vi "Measurement UI.vi"() -> ()   [LabVIEW 2021, in "Single Tone No Gen_Class D Amplifier_UI.lvlib"]
uses:
  Single Tone No Gen_Class D Amplifier_UI.lvlib
  shared/controls/units - snr.ctl
  shared/controls/units - ratio.ctl
  shared/ui/controls/view.ctl
  UI State.ctl
  <vilib>/Utility/miscctls.llb/LVBoundsTypeDef.ctl
  <vilib>/Utility/miscctls.llb/LVPoint32TypeDef.ctl
  <vilib>/Utility/miscctls.llb/LVPointTypeDef.ctl
  shared/ui/UI Helpers.lvlib
  shared/controls/audio controls.lvlib
panel:
  in  "view legend":T1
  out "time domain":waveform(dbl)[](graph)
  out "frequency domain":cluster{"x0":dbl, "dx":dbl, "magnitude":dbl[]}[](graph)
  out "meas table":string[][](table)
  out "output power (W)":dbl[](array[numeric])
  out "SFDR (dBc)":dbl[](array[numeric])
  out "gain":dbl[](array[numeric])
  out "dynamic range (dB)":dbl[](array[numeric])
  out "THD":dbl[](array[numeric])
  out "THD+N":dbl[](array[numeric])
  out "SNR":dbl[](array[numeric])
  out "phase (deg)":dbl[](array[numeric])
  out "amplitude (dBFS)":dbl[](array[numeric])
  out "amplitude (Vrms)":dbl[](array[numeric])
  out "frequency (Hz)":dbl[](array[numeric])
  out "channel names":string[](array[string])
  in  "Configuration tab":enum32{"Measurement", "Units"}(tab)
  in  "expected amplitude (Vpk)":dbl=1000.0 caption="Expected amplitude" format="%#_6f Vpk"
  in  "min settling cycles":u32 caption="Minimum settling cycles"
  in  "min settling time (s)":dbl=0.1 caption="Minimum settling time" format="%#_6ps"
  in  "min measurement cycles":u32 caption="Minimum measurement cycles"
  in  "min measurement time (s)":dbl=0.1 caption="Minimum measurement time" format="%#_6ps"
  in  "Acquisition channel":tag
  in  "acq sampling rate":dbl=51200.0 caption="Sample rate" format="%#.6pHz"
  in  "lowpass filter":T2(ring) caption="Lowpass filter"
  in  "highpass filter":enum32{"DC", "AC"}(ring) caption="Highpass filter"
  in  "band start":dbl=20.0 caption="Band start" format="%#_6pHz"
  in  "band stop":dbl=20000.0 caption="Band stop" format="%#_6pHz"
  in  "weighting filter":T3(ring)=enum."A-weighting" caption="Weighting filter"
  in  "load impedance":dbl=4.0 caption="Load impedance" format="%#_6p Ohms"
  in  "amplitude reference (Vpk-pk)":dbl=15.0 caption="Amplitude reference" format="%.3p Vpk-pk"
  in  "signal frequency":dbl=1000.0 caption="Estimated frequency" format="%#_6pHz"
  in  "gain units":T4 caption="Gain"
  in  "THD units":T4 caption="THD"
  in  "THD+N units":T4 caption="THD+N"
  in  "SNR units":T5 caption="SNR"
  in  "channel 0 offset":u32=1
  out "fft - data":dbl[](array[numeric])
  out "fft - df":dbl
  out "fft - f0":dbl
  out "wfm - data":dbl[](array[numeric])
  out "wfm - dt":dbl
  out "wfm - t0":dbl
  in  "acq channel":string="PXI1Slot4/ai0"
  in  "signal phase":dbl caption="phase"
  # "hidden controls - used to sync with MeasLink"
  # "hidden indicators"
  # "Filters"
  # "Acquisition"
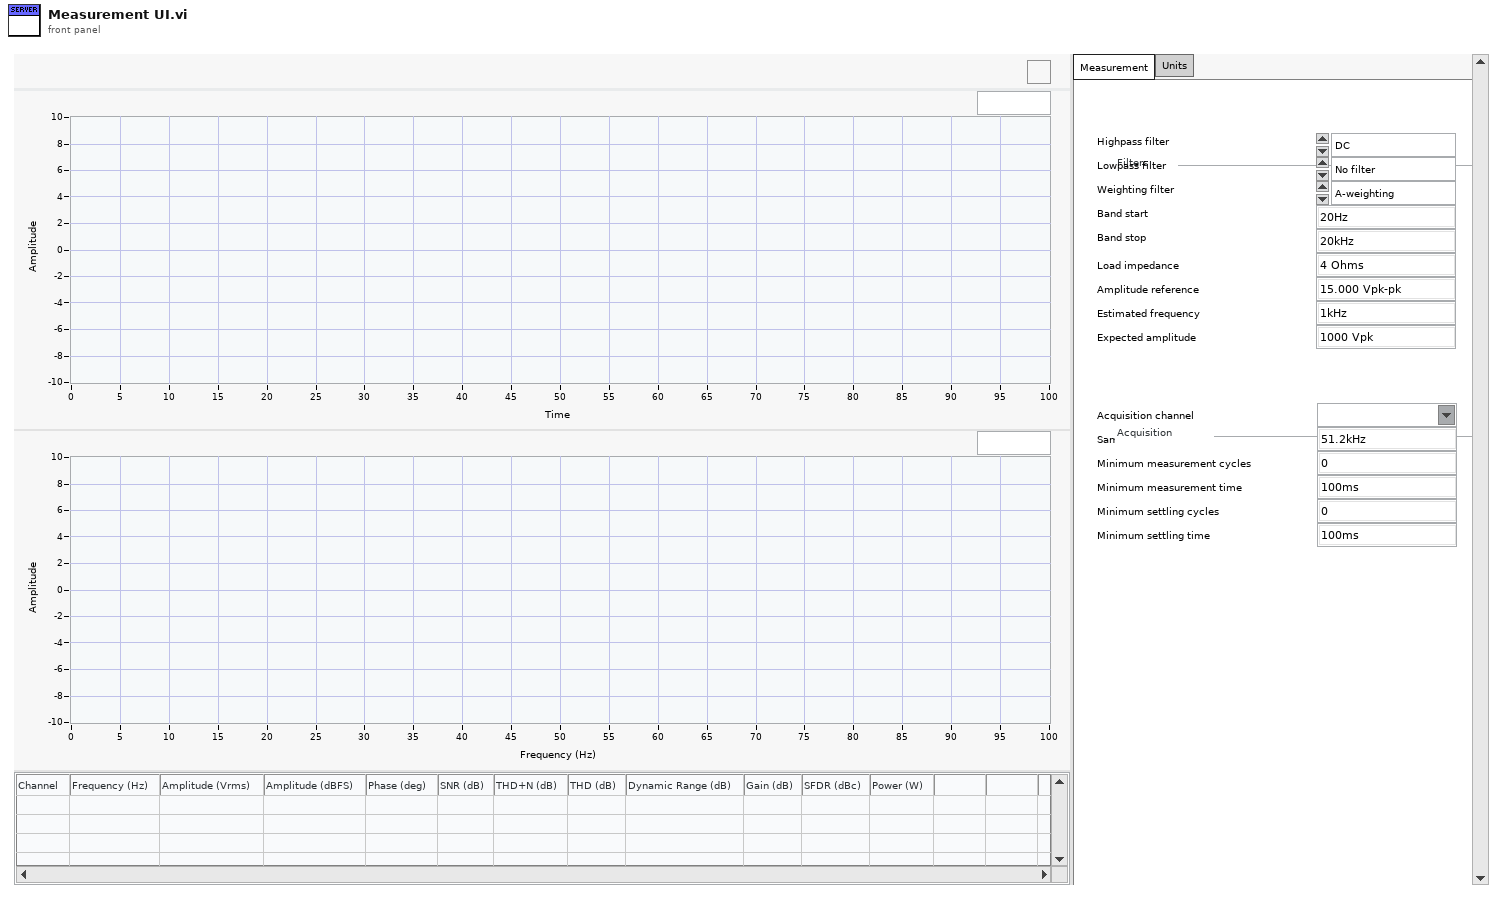
[diagram p1: front panel]
types:
  T1 = typedef "UI Helpers.lvlib/view.ctl" = bool
  T2 = enum32{"No filter", "AES17 20kHz", "AES17 40kHz"}
  T3 = enum32{"Linear", "A-weighting", "B-weighting", "C-weighting"}
  T4 = typedef "audio controls.lvlib/units - ratio.ctl" = enum32{"dB", "%", "x/y"}
  T5 = typedef "audio controls.lvlib/units - snr.ctl" = enum32{"dB", "x/y"}
  T6 = typedef "LVPointTypeDef.ctl" = cluster{"Horizontal":i16, "Vertical":i16}
  T7 = typedef "Single Tone No Gen_Class D Amplifier_UI.lvlib/UI State.ctl" = cluster{"Graph Size":T8, "Legend Visible":bool, "Mouse Coords":T9, "Show All Plots":bool}
  T8 = typedef "LVBoundsTypeDef.ctl" = cluster{"Width":u32, "Height":u32}
  T9 = typedef "LVPoint32TypeDef.ctl" = cluster{"Horizontal":i32, "Vertical":i32}
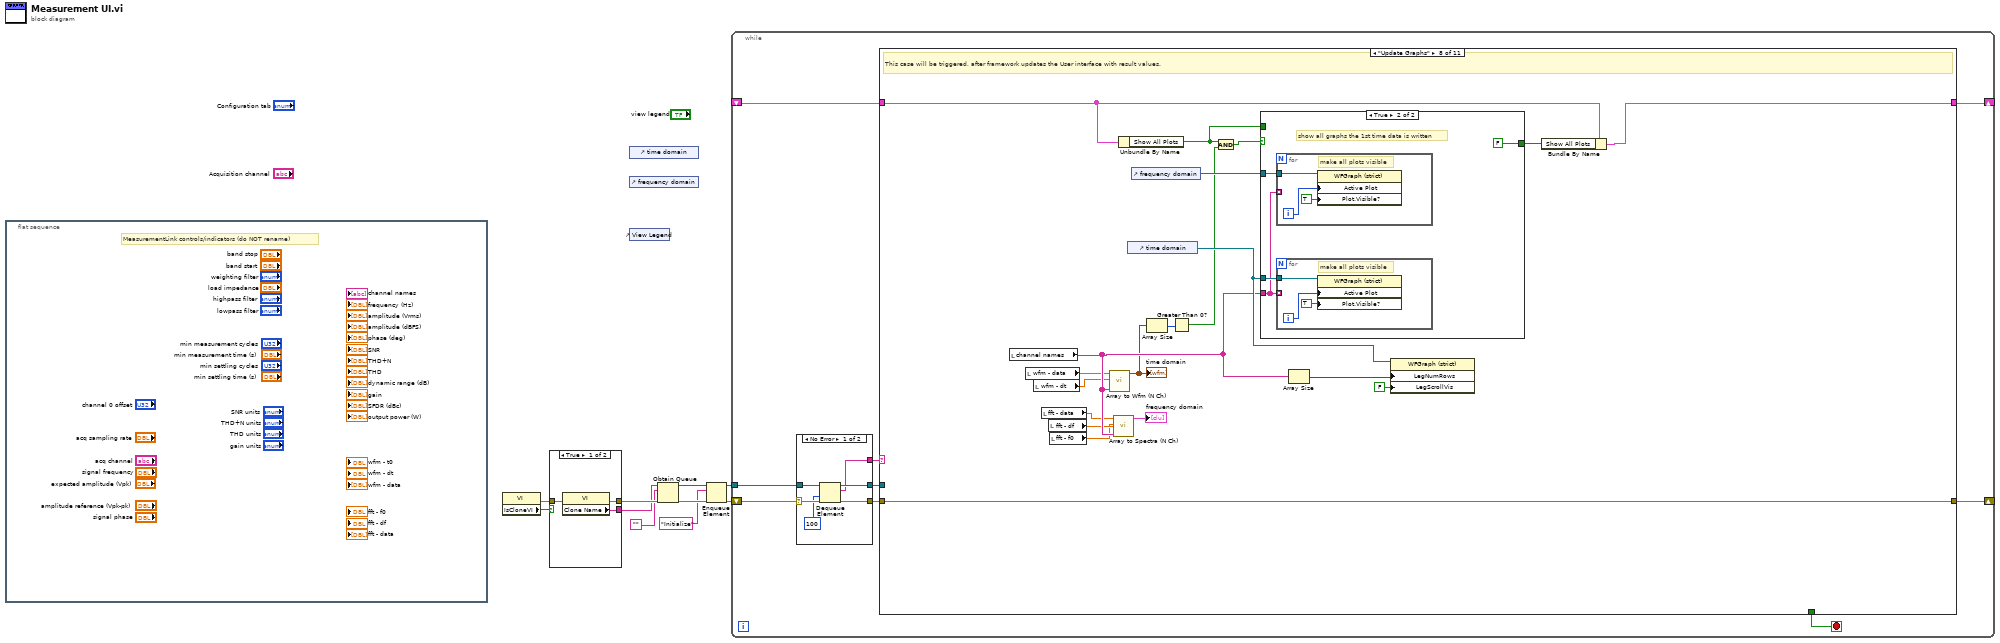
[diagram p0: block diagram]
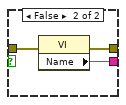
[diagram p2: hidden frame]
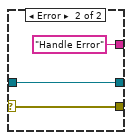
[diagram p3: hidden frame]
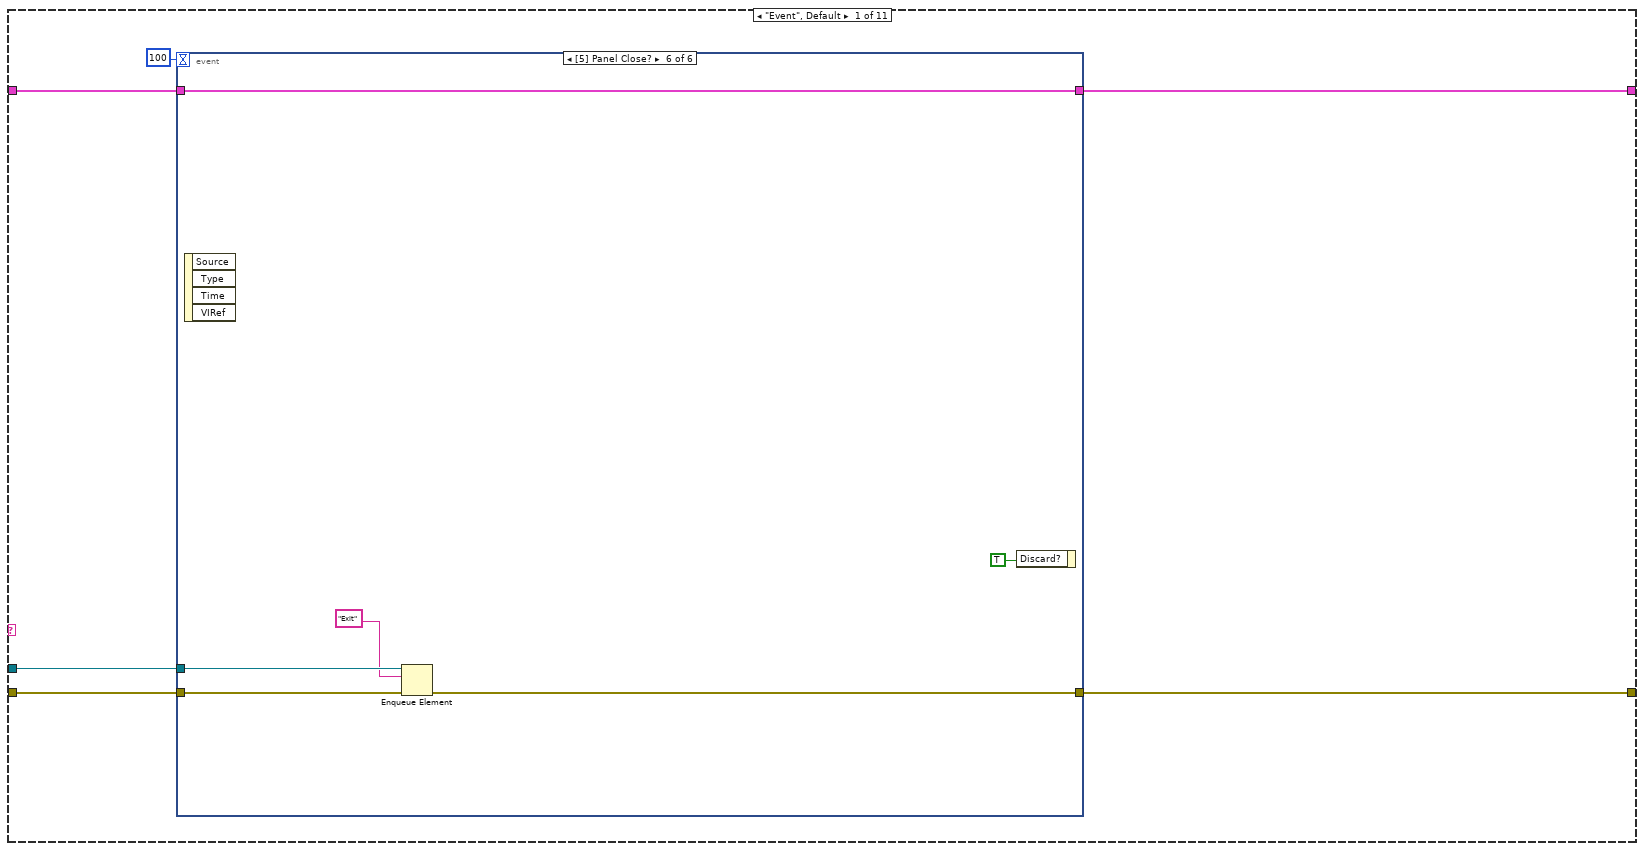
[diagram p4: hidden frame]
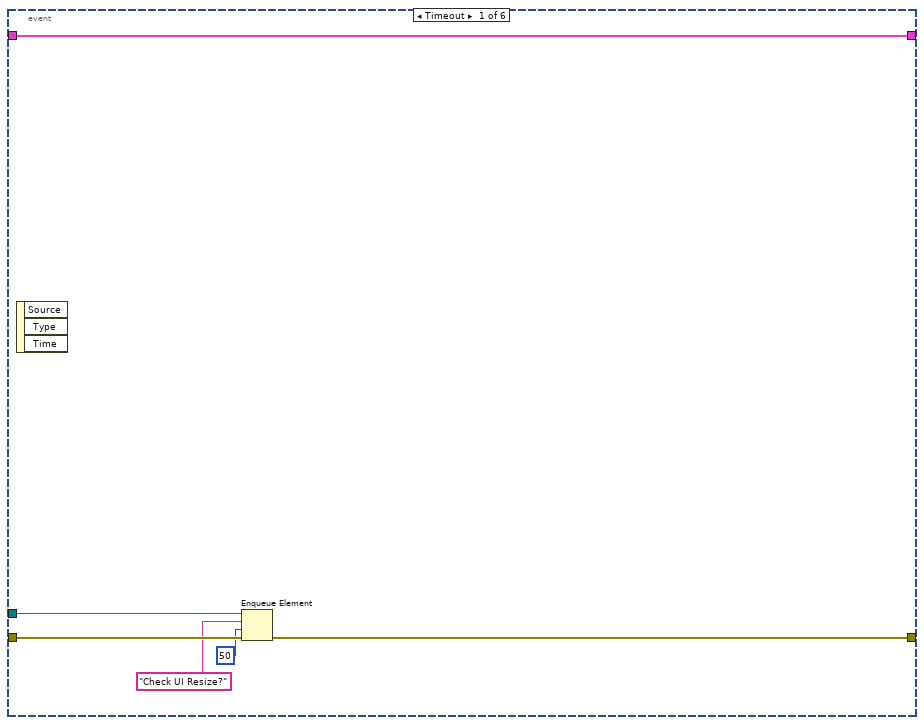
[diagram p5: hidden frame]
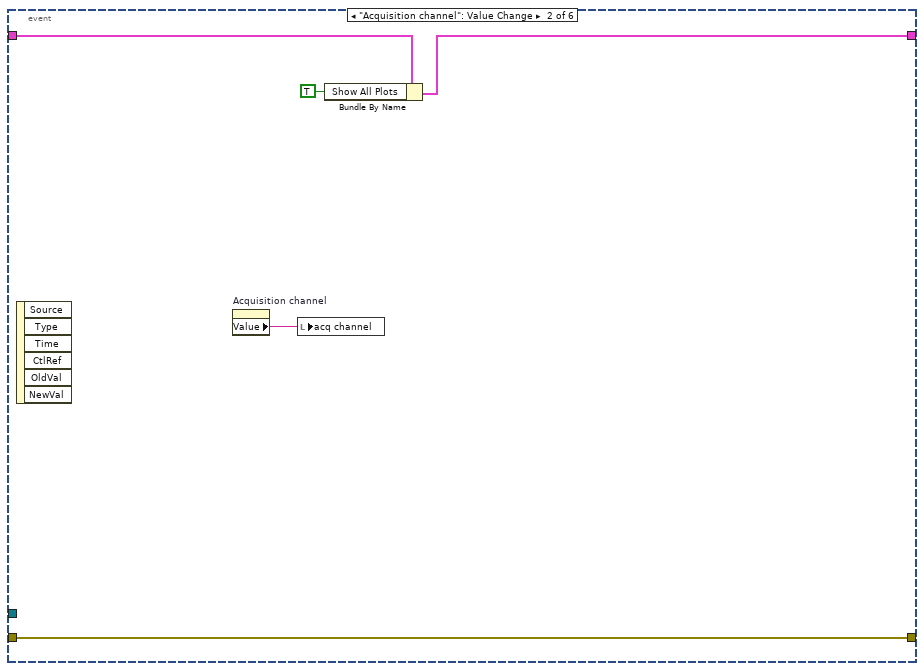
[diagram p6: hidden frame]
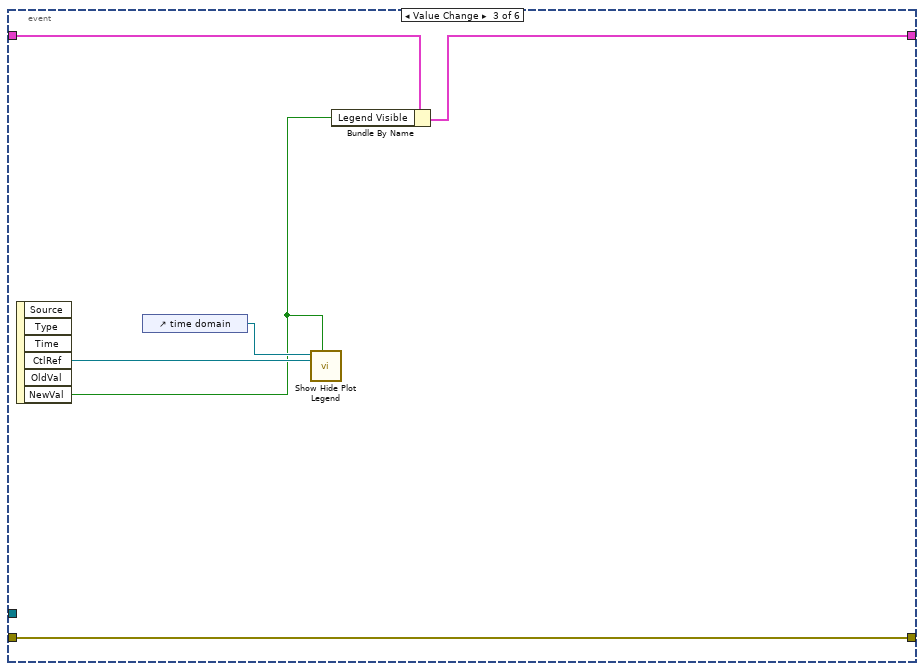
[diagram p7: hidden frame]
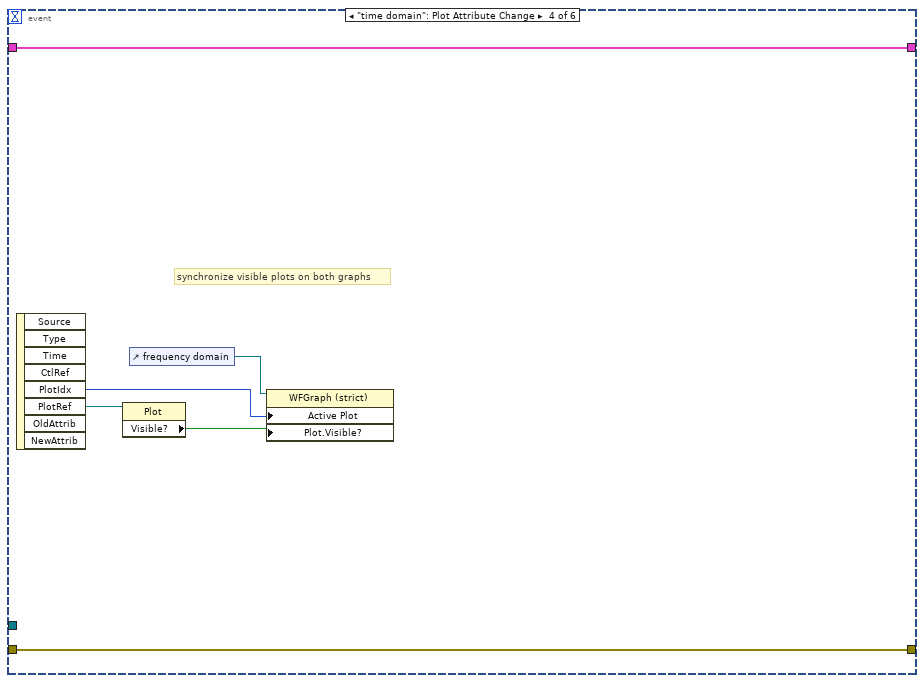
[diagram p8: hidden frame]
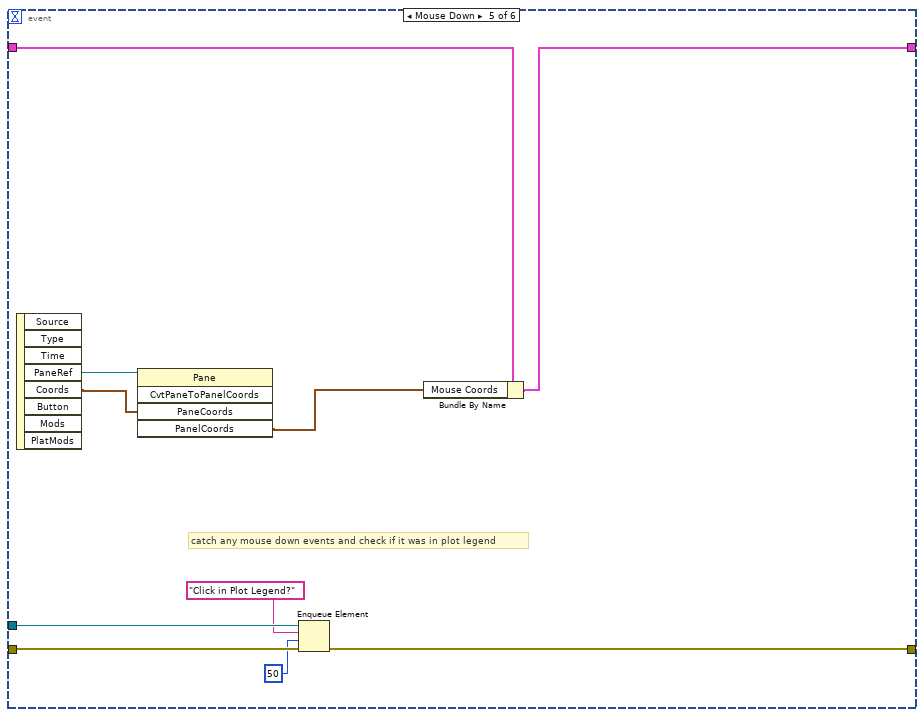
[diagram p9: hidden frame]
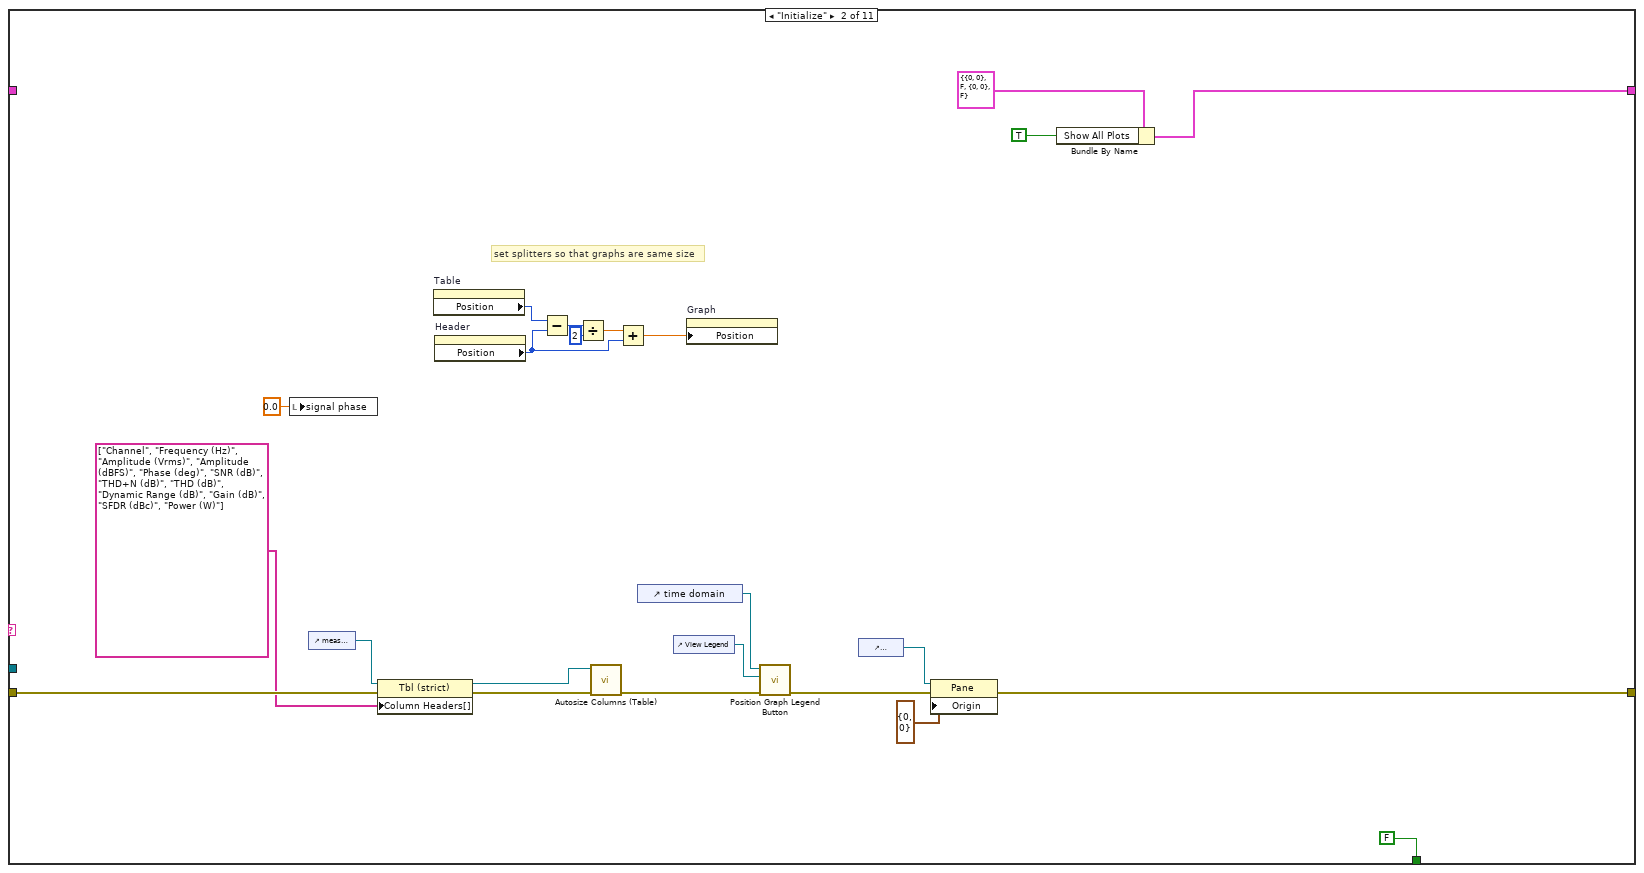
[diagram p10: hidden frame]
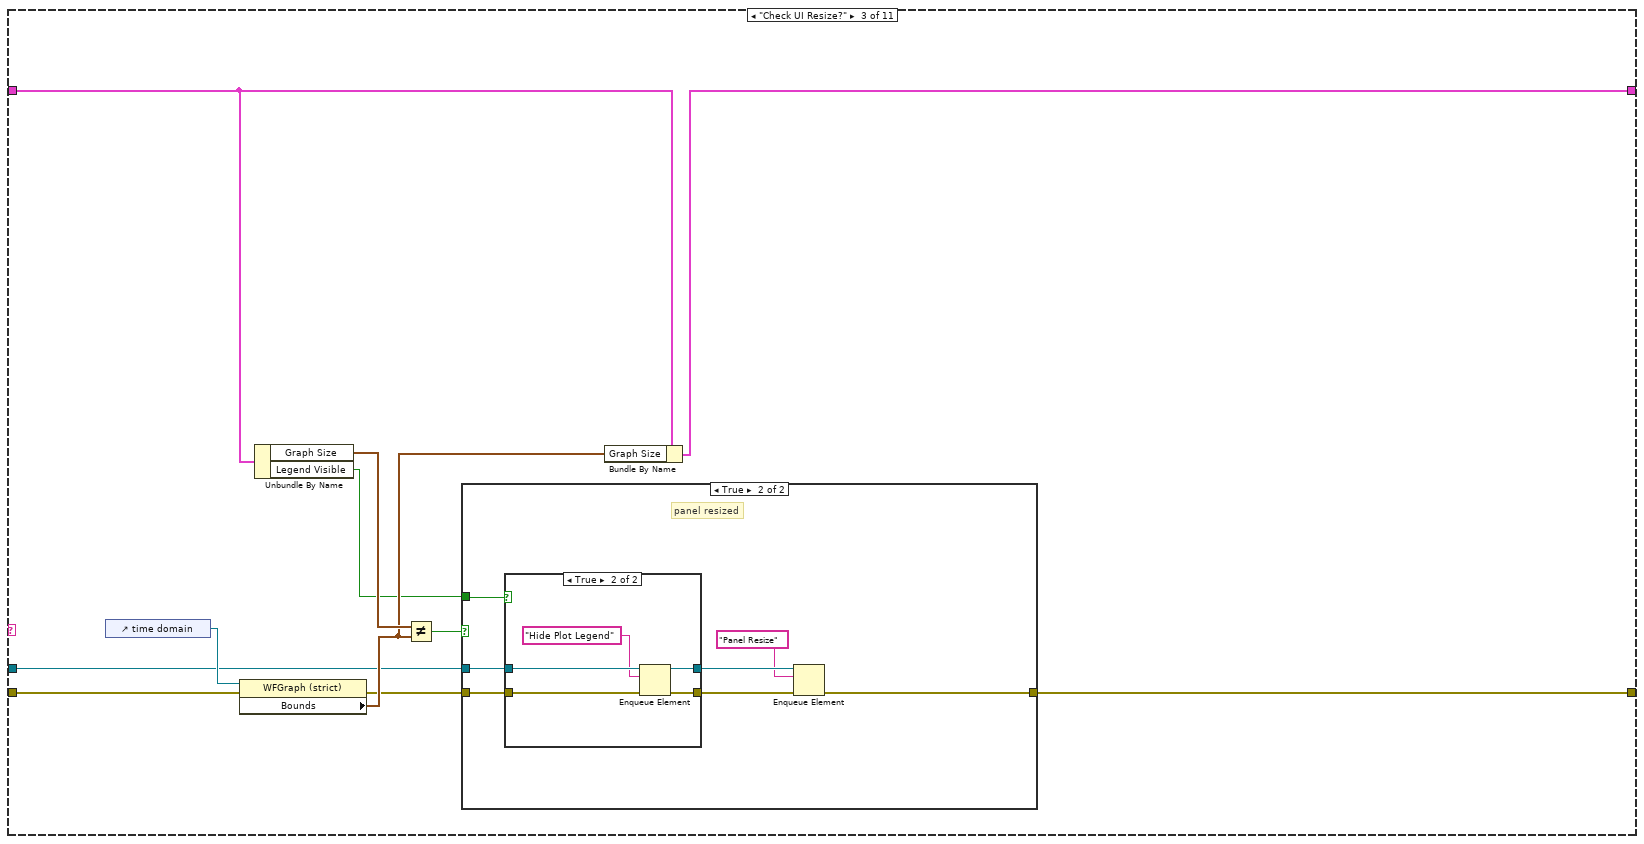
[diagram p11: hidden frame]
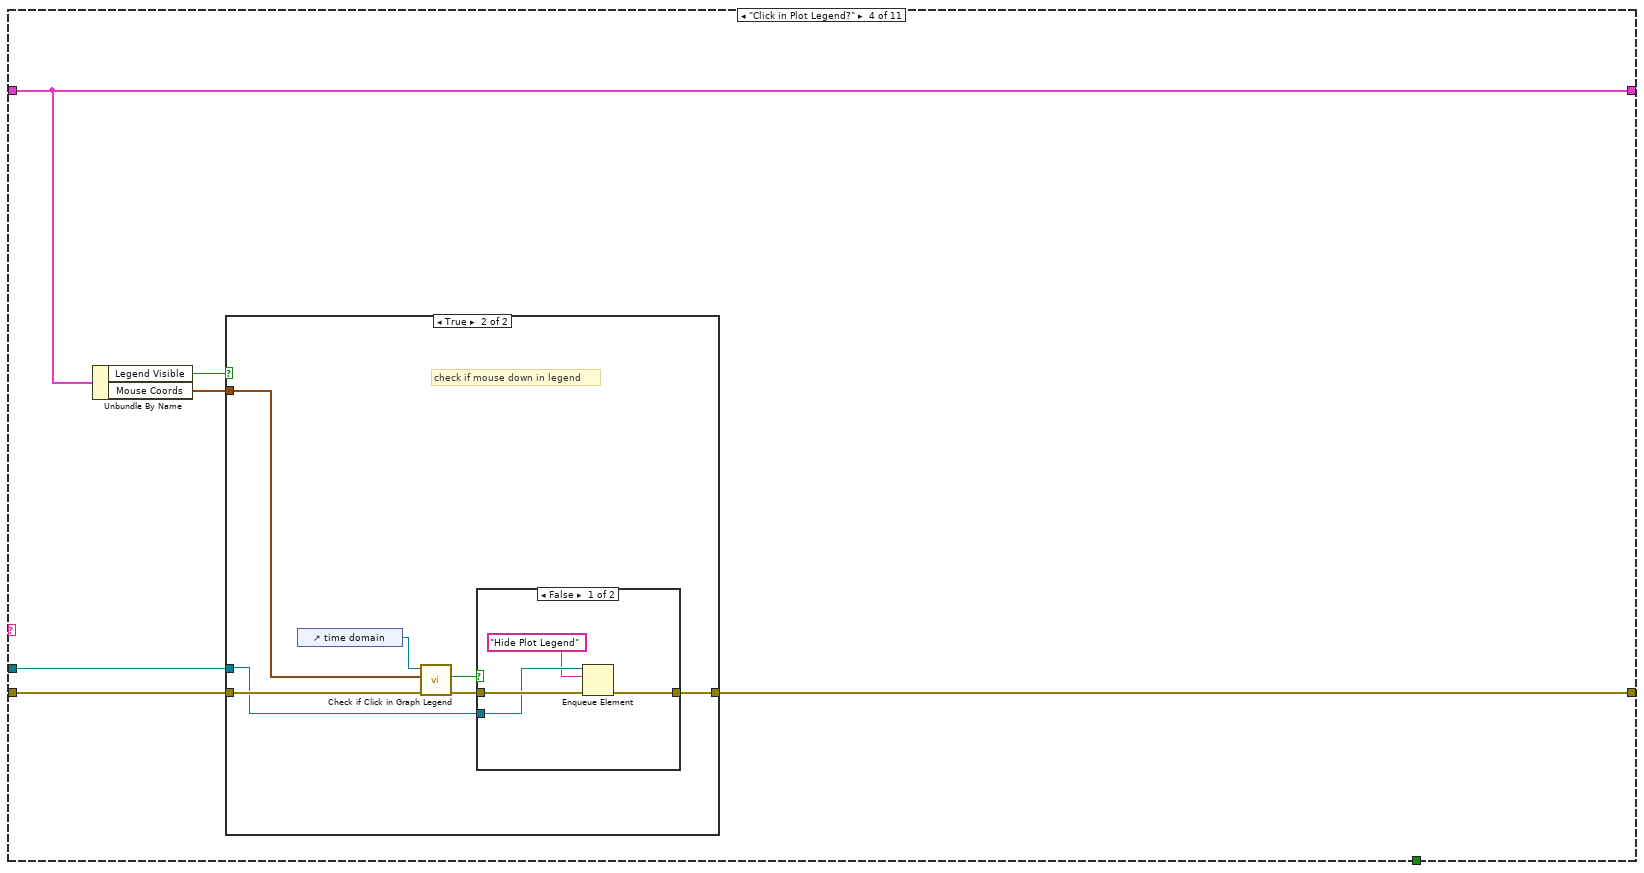
[diagram p14: hidden frame]
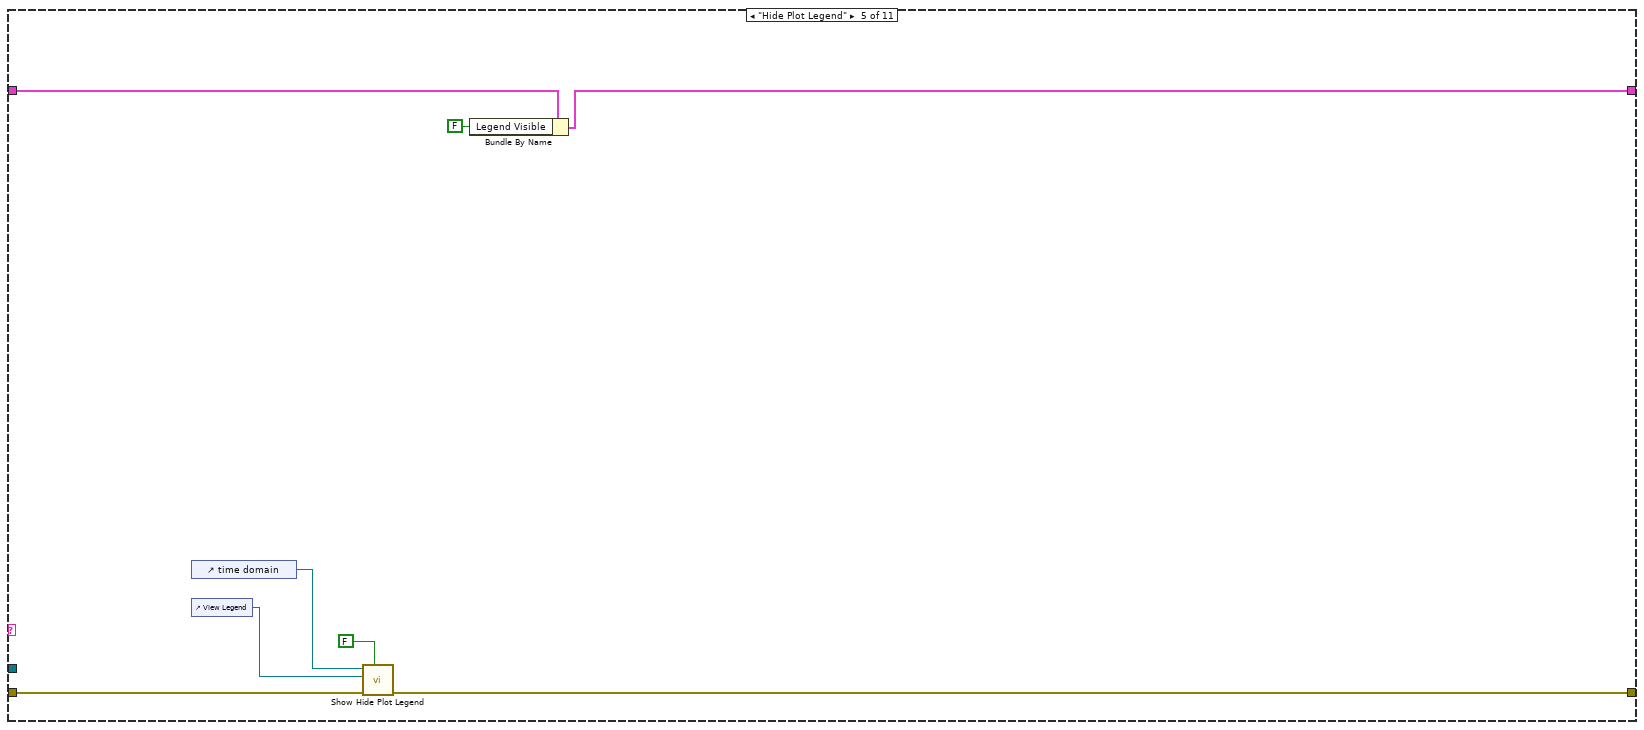
[diagram p17: hidden frame]
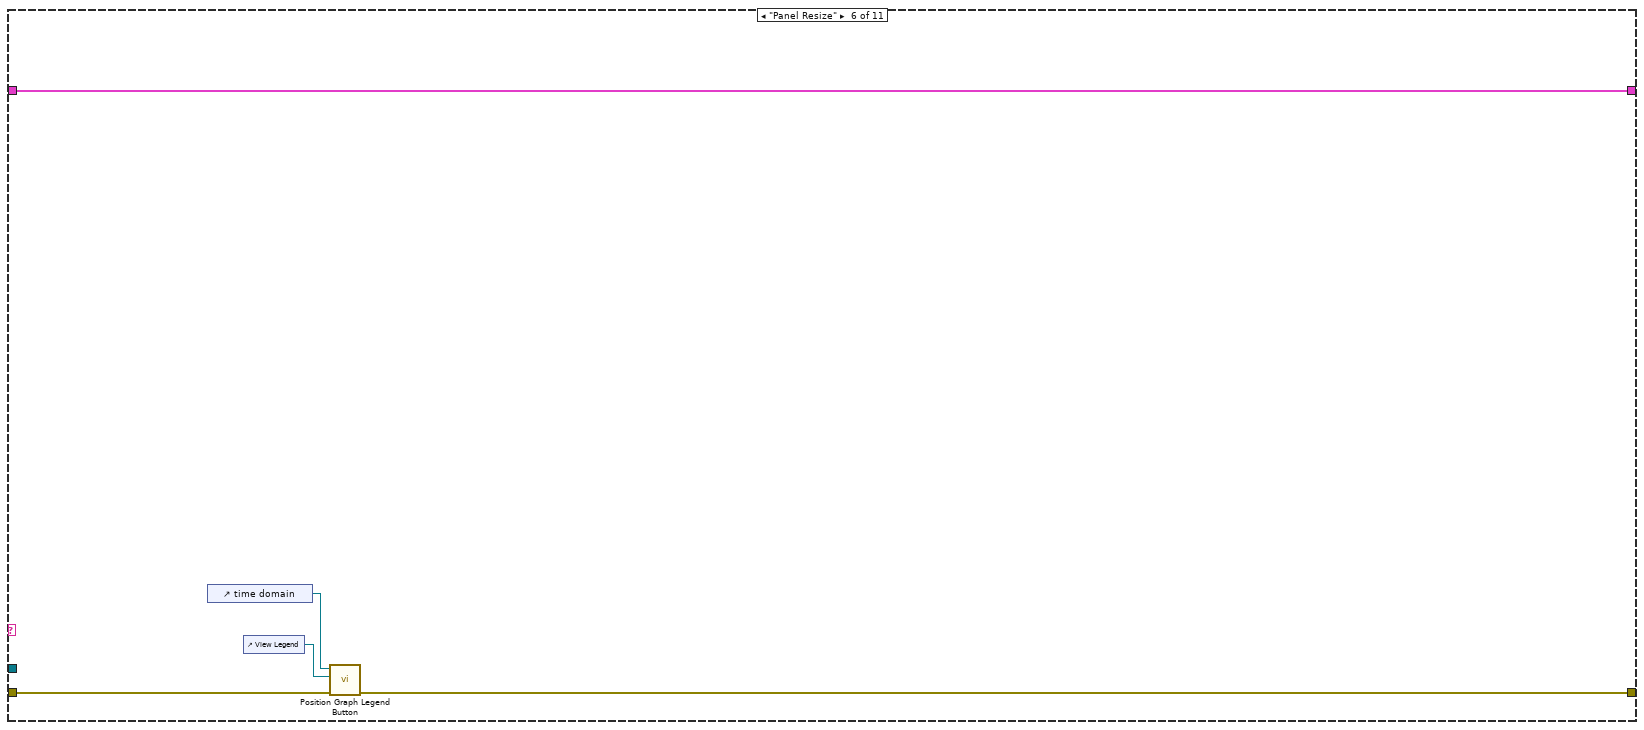
[diagram p18: hidden frame]
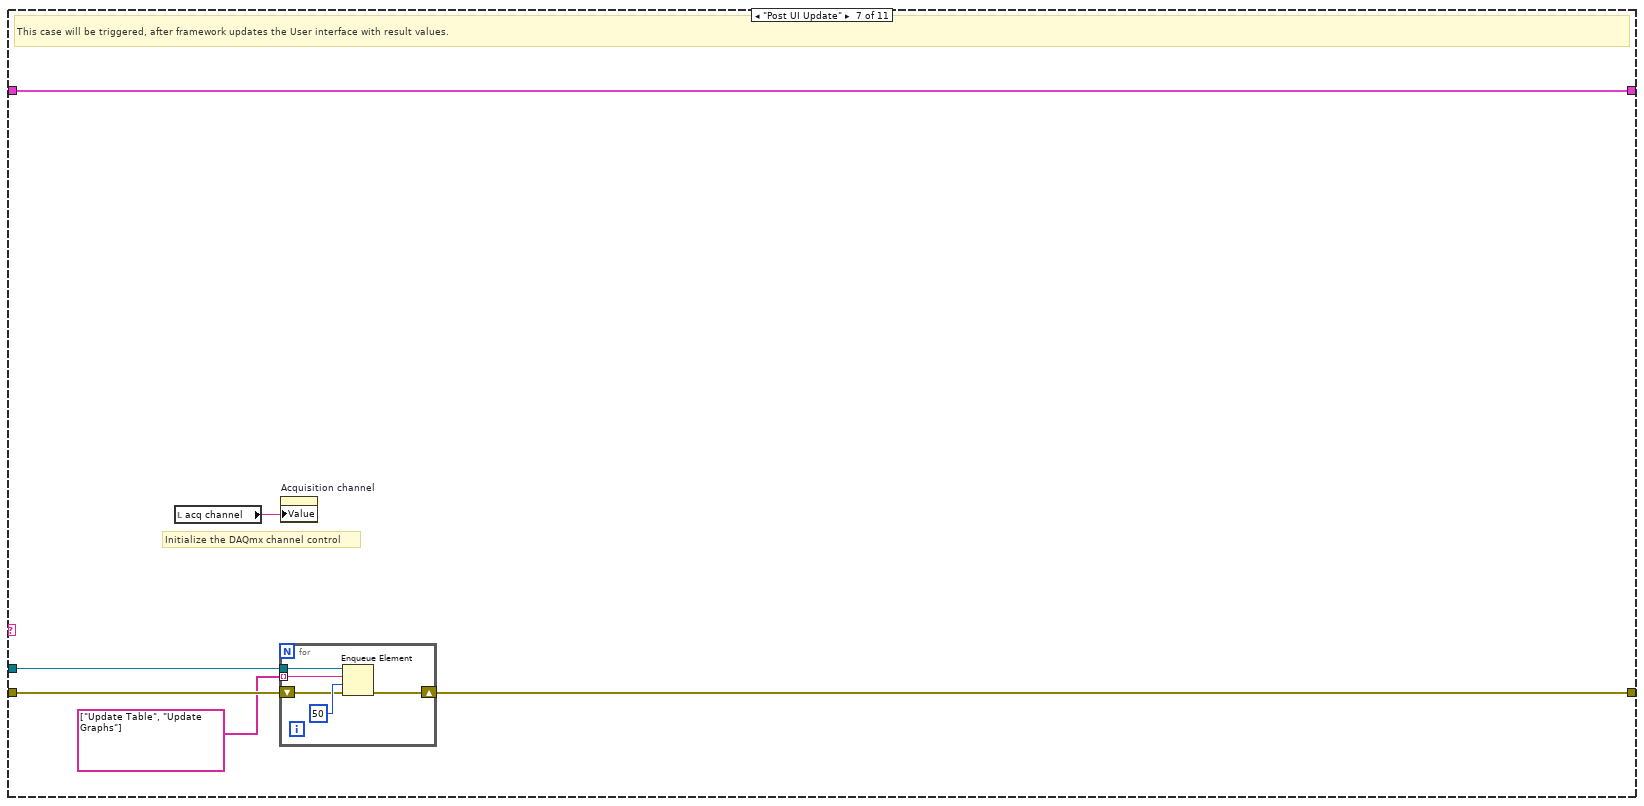
[diagram p19: hidden frame]
diagram:
  n1 = flat-sequence {
    frame #0 {
      # "MeasurementLink controls/indicators (do NOT rename)"
    }
  }
  n2 = property class="VI"() -> (error out=w1:errorcluster, "IsCloneVI"=w2:bool)  [unwired: 2 in, 1 out]
  n3 = case shown="True" w2 {
    tunnel: [w13 w16] -> w10
    tunnel: [w12 w15] -> w9
    tunnel: w1 -> [w11 w14]
    frame True {
      n4 = property class="VI"(error in=w11) -> (error out=w13:errorcluster, "Clone Name"=w12:string)  [unwired: 1 in, 1 out]
    }
    frame False {
      n5 = property class="VI"(error in=w14) -> (error out=w16:errorcluster, "Name"=w15:string)  [unwired: 1 in, 1 out]
    }
  }
  n6 = control-ref of="time domain"() -> ()  [unwired: 1 out]
  n7 = control-ref of="frequency domain"() -> ()  [unwired: 1 out]
  n8 = control-ref of="View Legend"() -> ()  [unwired: 1 out]
  n9 = Obtain Queue(name (unnamed)=w9, element data type="", error in (no error)=w10) -> (queue out=w6:refnum<queue>, error out=w8:errorcluster)  [unwired: 2 in, 1 out]
  n10 = Enqueue Element(queue=w6, element="Initialize", error in (no error)=w8) -> (queue out=w5:refnum<queue>, error out=w7:errorcluster)  [unwired: 1 in, 1 out]
  n11 = while {
    shift-right: [w20] -> _
    shift-left: w7 -> [w25]
    tunnel: w5 -> [w23]
    shift-right: [w18] -> _
    shift-left: _ -> [w17]
    stop <- w19 stop-if-true
    n12 = case shown="No Error" w25 {
      selector: w25 -> [w31 w34]
      tunnel: [w30 w34] -> w24
      tunnel: w23 -> [w29 w33]
      tunnel: [w28 w33] -> w22
      tunnel: [w27 "Handle Error"] -> w21
      frame No Error {
        n13 = Dequeue Element(queue=w29, timeout in ms (-1)=100, error in (no error)=w31) -> (queue out=w28:refnum<queue>, element=w27:string, error out=w30:errorcluster)  [unwired: 1 out]
      }
      frame Error {
      }
    }
    n14 = case shown="\"Update Graphs\"" w21 {
      tunnel: w24 -> [w39 w97 w112 w130 w152 w157 w164 w191 w203 w329 w331]
      tunnel: w22 -> [w37 _ w103 w131 _ _ w163 _ _ w327 _]
      tunnel: [w40 w80 w105 w129 w151 w156 w161 w191 w207 w324 w331] -> w20
      tunnel: [_ FALSE _ _ _ _ _ _ _ TRUE _] -> w19
      tunnel: [w35 w85 w108 w134 w153 w160 w165 w183 w204 w322 w330] -> w18
      tunnel: w17 -> [w36 _ w109 w134 w154 w160 w165 w184 w204 w322 w330]
      frame "Event", Default {
        n15 = event shown="[5] Panel Close?" {
          selector: _ -> [_ _ _ _ _ _]
          dyn-events: _ -> [_ _ _ _ _ _]
          timeout: 100 -> [_ _ _ _ _ _]
          tunnel: [w43 w50 w54 w58 w71 w77] -> w40
          tunnel: w39 -> [w46 w50 w54 w58 w72 w78]
          tunnel: w37 -> [w45 _ _ _ w73 w76]
          tunnel: w36 -> [w42 w49 w56 w59 w68 w74]
          tunnel: [w42 w48 w55 w59 w67 w74] -> w35
          event Timeout {
            n16 = event-data() -> ()  [unwired: 1 in, 3 out]
            n17 = Enqueue Element(queue=w45, element="Check UI Resize?", timeout in ms (-1)=50, error in (no error)=w46) -> (error out=w43:errorcluster)  [unwired: 2 out]
          }
          event "Acquisition channel": Value Change {
            n18 = event-data() -> ()  [unwired: 1 in, 6 out]
            n19 = property on="Acquisition channel" class="DAQmxName"() -> ("Value"=w51:string)  [unwired: 2 in, 2 out]
            n20 = local write "acq channel"(w51) -> ()
            n21 = Bundle By Name(cluster=w49, "Show All Plots"=TRUE) -> (w48:T7)
          }
          event Value Change {
            n22 = event-data() -> ("CtlRef"=w53:refnum<vi>, "NewVal"=w52:T1)  [unwired: 1 in, 4 out]
            n23 = control-ref of="time domain"() -> (w57:refnum<vi>)
            n24 = call "Show Hide Plot Legend.vi"("show"=w52, "view reference"=w53, "graph reference"=w57) -> ()  [unwired: 8 in, 1 out]
            n25 = Bundle By Name(cluster=w56, "Legend Visible"=w52) -> (w55:T7)
          }
          event "time domain": Plot Attribute Change {
            # "synchronize visible plots on both graphs"
            n26 = event-data() -> ("PlotIdx"=w61:i32, "PlotRef"=w62:refnum<vi>)  [unwired: 1 in, 6 out]
            n27 = property class="Plot"(reference=w62) -> ("Visible?"=w63:bool)  [unwired: 1 in, 2 out]
            n28 = control-ref of="frequency domain"() -> (w60:refnum<vi>)
            n29 = property on="Property Node" class="WFGraph (strict)"(reference=w60, "Active Plot"=w61, "Plot.Visible?"=w63) -> ()  [unwired: 1 in, 2 out]
          }
          event Mouse Down {
            # "catch any mouse down events and check if it was in plot legend"
            n30 = event-data() -> ("PaneRef"=w66:refnum<vi>, "Coords"=w65:T9)  [unwired: 1 in, 6 out]
            n31 = invoke class="Pane" method="CvtPaneToPanelCoords"(reference=w66, "PaneCoords"=w65) -> ("PanelCoords"=w64:T6)  [unwired: 3 in, 4 out]
            n32 = Enqueue Element(queue=w73, element="Click in Plot Legend?", timeout in ms (-1)=50, error in (no error)=w72) -> (error out=w71:errorcluster)  [unwired: 2 out]
            n33 = Bundle By Name(cluster=w68, "Mouse Coords"=w64) -> (w67:T7)
          }
          event Panel Close? {
            n34 = event-data() -> ()  [unwired: 1 in, 4 out]
            n35 = Enqueue Element(queue=w76, element="Exit", error in (no error)=w78) -> (error out=w77:errorcluster)  [unwired: 1 in, 2 out]
            n36 = event-data("Discard?"=TRUE) -> ()  [unwired: 1 in, 1 out]
          }
        }
      }
      frame "Initialize" {
        # "set splitters so that graphs are same size"
        n37 = local write "signal phase"(0.0 ("signal phase")) -> ()
        n38 = control-ref of="meas table"() -> (w95:refnum<vi>)
        n39 = property class="Tbl (strict)"(reference=w95, error in=w97, "Column Headers[]"=string[] ["Channel", "Frequency (Hz)", "Amplitude (Vrms)", "Amplitude (dBFS)", "Phase (deg)", "SNR (dB)", "THD+N (dB)", "THD (dB)", "Dynamic Range (dB)", "Gain (dB)", "SFDR (dBc)", "Power (W)"] ("Column Header Strings[]")) -> (reference out=w94:refnum<vi>, error out=w96:errorcluster)
        n40 = property on="Table" class="Splitter"() -> ("Position"=w92:i32)  [unwired: 2 in, 2 out]
        n41 = property on="Header" class="Splitter"() -> ("Position"=w88:i32)  [unwired: 2 in, 2 out]
        n42 = Subtract(x=w92, y=w88) -> (x-y=w91:i32)
        n43 = Divide(x=w91, y=2) -> (x/y=w89:dbl)
        n44 = call "Autosize Columns (Table).vi"("error in (no error)"=w96, "table"=w94) -> ("error out"=w98:errorcluster)  [unwired: 9 in]
        n45 = Add(x=w89, y=w88) -> (x+y=w87:dbl)
        n46 = control-ref of="time domain"() -> (w100:refnum<vi>)
        n47 = control-ref of="View Legend"() -> (w99:refnum<vi>)
        n48 = property on="Graph" class="Splitter"("Position"=w87) -> ()  [unwired: 2 in, 2 out]
        n49 = call "Position Graph Legend Button.vi"("error in (no error)"=w98, "view legend"=w99, "graph"=w100) -> ("error out"=w83:errorcluster)  [unwired: 8 in]
        n50 = control-ref of="Configuration"() -> (w82:refnum<vi>)
        n51 = property class="Pane"(reference=w82, error in=w83, "Origin"=T6 {"Horizontal"=0, "Vertical"=0}) -> (error out=w80:errorcluster)  [unwired: 1 out]
        n52 = Bundle By Name(cluster=T7 {"Graph Size"={"Width"=0, "Height"=0}, "Legend Visible"=FALSE, "Mouse Coords"={"Horizontal"=0, "Vertical"=0}, "Show All Plots"=FALSE} ("ui state"), "Show All Plots"=TRUE ("Init Graph Plot Legend")) -> (w85:T7)
      }
      frame "Check UI Resize?" {
        n53 = control-ref of="time domain"() -> (w113:refnum<vi>)
        n54 = property on="Property Node" class="WFGraph (strict)"(reference=w113, error in=w112) -> (error out=w106:errorcluster, "Bounds"=w110:T8)  [unwired: 1 out]
        n55 = Unbundle By Name(w109) -> ("Graph Size"=w111:T8, "Legend Visible"=w104:bool)
        n56 = Not Equal?(x=w111, y=w110) -> (x != y?=w107:bool)
        n57 = case shown="True" w107 {
          tunnel: w106 -> [w114 w121]
          tunnel: [w114 w116] -> w105
          tunnel: w104 -> [_ w119]
          tunnel: w103 -> [_ w120]
          frame False {
            # "no resize"
          }
          frame True {
            # "panel resized"
            n58 = case shown="True" w119 {
              tunnel: w121 -> [w123 w128]
              tunnel: [w123 w127] -> w118
              tunnel: w120 -> [w122 w126]
              tunnel: [w122 w124] -> w117
              frame False {
              }
              frame True {
                n59 = Enqueue Element(queue=w126, element="Hide Plot Legend", error in (no error)=w128) -> (queue out=w124:refnum<queue>, error out=w127:errorcluster)  [unwired: 1 in, 1 out]
              }
            }
            n60 = Enqueue Element(queue=w117, element="Panel Resize", error in (no error)=w118) -> (error out=w116:errorcluster)  [unwired: 1 in, 2 out]
          }
        }
        n61 = Bundle By Name(cluster=w109, "Graph Size"=w110) -> (w108:T7)
      }
      frame "Click in Plot Legend?" {
        n62 = Unbundle By Name(w134) -> ("Legend Visible"=w133:bool, "Mouse Coords"=w132:T9)
        n63 = case shown="True" w133 {
          tunnel: w132 -> [_ w140]
          tunnel: w131 -> [_ w137]
          tunnel: w130 -> [w135 w142]
          tunnel: [w135 w136] -> w129
          frame False {
            # "legend not visible; do nothing"
          }
          frame True {
            # "check if mouse down in legend"
            n64 = control-ref of="time domain"() -> (w141:refnum<vi>)
            n65 = call "Check if Click in Graph Legend.vi"("error in (no error)"=w142, "Mouse Coords"=w140, "WaveformGraph"=w141) -> ("error out"=w138:errorcluster, "click in legend?"=w139:bool)  [unwired: 7 in]
            n66 = case shown="False" w139 {
              tunnel: w138 -> [w146 w147]
              tunnel: w137 -> [w145 _]
              tunnel: [w144 w147] -> w136
              frame False {
                n67 = Enqueue Element(queue=w145, element="Hide Plot Legend", error in (no error)=w146) -> (error out=w144:errorcluster)  [unwired: 1 in, 2 out]
              }
              frame True {
                # "inside legend; do nothing"
              }
            }
          }
        }
      }
      frame "Hide Plot Legend" {
        n68 = control-ref of="time domain"() -> (w149:refnum<vi>)
        n69 = control-ref of="View Legend"() -> (w148:refnum<vi>)
        n70 = call "Show Hide Plot Legend.vi"("show"=FALSE, "error in (no error)"=w152, "view reference"=w148, "graph reference"=w149) -> ("error out"=w151:errorcluster)  [unwired: 7 in]
        n71 = Bundle By Name(cluster=w154, "Legend Visible"=FALSE ("legend visible")) -> (w153:T7)
      }
      frame "Panel Resize" {
        n72 = control-ref of="time domain"() -> (w159:refnum<vi>)
        n73 = control-ref of="View Legend"() -> (w158:refnum<vi>)
        n74 = call "Position Graph Legend Button.vi"("error in (no error)"=w157, "view legend"=w158, "graph"=w159) -> ("error out"=w156:errorcluster)  [unwired: 8 in]
      }
      frame "Post UI Update" {
        # "Initialize the DAQmx channel control"
        # "This case will be triggered, after framework updates the User interface with result values."
        n75 = local read "acq channel"() -> (w166:string)
        n76 = for {
          tunnel: w163 -> [w169]
          shift-right: [w168] -> w161
          shift-left: w164 -> [w170]
          tunnel: string[] ["Update Table", "Update Graphs"] -> [w167] mode=indexing
          n77 = Enqueue Element(queue=w169, element=w167, timeout in ms (-1)=50, error in (no error)=w170) -> (error out=w168:errorcluster)  [unwired: 2 out]
        }
        n78 = property on="Acquisition channel" class="DAQmxName"("Value"=w166) -> ()  [unwired: 2 in, 2 out]
      }
      frame "Update Graphs" {
        # "This case will be triggered, after framework updates the User interface with result values."
        n79 = local read "channel names"() -> (w187:string[])
        n80 = local read "wfm - data"() -> (w182:dbl[])
        n81 = local read "wfm - dt"() -> (w181:dbl)
        n82 = local read "fft - data"() -> (w180:dbl[])
        n83 = local read "fft - df"() -> (w179:dbl)
        n84 = local read "fft - f0"() -> (w178:dbl)
        n85 = call "Array to Wfm (N Ch).vi"("channel names"=w187, "dt"=w181, "array"=w182) -> ("waveforms"=w176:waveform(dbl)[])  [unwired: 8 in]
        "time domain" <- w176
        n86 = call "Array to Spectra (N Ch).vi"("channel names"=w187, "df"=w179, "f0"=w178, "data"=w180) -> ("spectra"=→"frequency domain":cluster{"f0":dbl, "df":dbl, "data":dbl[]}[])  [unwired: 7 in]
        n87 = Unbundle By Name(w184) -> ("Show All Plots"=w172:bool)
        n88 = control-ref of="time domain"() -> (w190:refnum<vi>)
        n89 = control-ref of="frequency domain"() -> (w186:refnum<vi>)
        n90 = Array Size(array=w176) -> (size(s)=w175:i32)
        n91 = Greater Than 0?(x=w175) -> (x > 0?=w174:bool)
        n92 = And(x=w172, y=w174) -> (x .and. y?=w173:bool)
        n93 = case shown="True" w173 {
          tunnel: w190 -> [_ w196]
          tunnel: w187 -> [_ w195]
          tunnel: w186 -> [_ w194]
          tunnel: [w192 FALSE] -> w185
          tunnel: w172 -> [w192 _]
          frame False {
          }
          frame True {
            # "show all graphs the 1st time data is written"
            n94 = for {
              tunnel: w194 -> [w197]
              tunnel: w195 -> [_] mode=indexing
              i -> [w198]
              # "make all plots visible"
              n95 = property class="WFGraph (strict)"(reference=w197, "Active Plot"=w198, "Plot.Visible?"=TRUE ("Plot.Visible")) -> ()  [unwired: 1 in, 2 out]
            }
            n96 = for {
              tunnel: w196 -> [w200]
              tunnel: w195 -> [_] mode=indexing
              i -> [w201]
              # "make all plots visible"
              n97 = property class="WFGraph (strict)"(reference=w200, "Active Plot"=w201, "Plot.Visible?"=TRUE ("Plot.Visible")) -> ()  [unwired: 1 in, 2 out]
            }
          }
        }
        n98 = Array Size(array=w187) -> (size(s)=w189:i32)
        n99 = property class="WFGraph (strict)"(reference=w190, "LegNumRows"=w189, "LegScrollVis"=FALSE ("Legend:Scrollbar Visible")) -> ()  [unwired: 1 in, 2 out]
        n100 = Bundle By Name(cluster=w184, "Show All Plots"=w185) -> (w183:T7)
      }
      frame "Update Table" {
        # "format data for table"
        # "This case will be triggered, after framework updates the User interface with result values."
        n101 = local read "SNR units"() -> (w247:T5)
        n102 = local read "THD+N units"() -> (w259:T4)
        n103 = local read "THD units"() -> (w245:T4)
        n104 = local read "gain units"() -> (w243:T4)
        n105 = case shown="\"x/y\"" w247 {
          tunnel: ["(dB)" "(ratio)"] -> w258
          tunnel: ["%5.1f" ("initial string") "%.1f" ("initial string")] -> w241
          frame "dB", Default {
          }
          frame "x/y" {
          }
        }
        n106 = case shown="\"x/y\"" w259 {
          tunnel: ["(dB)" "(%)" "(ratio)"] -> w261
          tunnel: ["%5.1f" ("initial string") "%.3f" ("initial string") "%.6f" ("initial string")] -> w238
          frame "dB", Default {
          }
          frame "%" {
          }
          frame "x/y" {
          }
        }
        n107 = case shown="\"x/y\"" w245 {
          tunnel: ["(dB)" "(%)" "(ratio)"] -> w246
          tunnel: ["%5.1f" ("initial string") "%.3f" ("initial string") "%.6f" ("initial string")] -> w235
          frame "dB", Default {
          }
          frame "%" {
          }
          frame "x/y" {
          }
        }
        n108 = case shown="\"%\"" w243 {
          tunnel: ["(dB)" "(%)" "(ratio)"] -> w244
          tunnel: ["%5.1f" ("initial string") "%.1f" ("initial string") "%.3f" ("initial string")] -> w225
          frame "dB", Default {
          }
          frame "%" {
          }
          frame "x/y" {
          }
        }
        n109 = Concatenate Strings("SNR " ("string"), w258) -> (w255:string)
        n110 = Concatenate Strings("THD+N " ("string"), w261) -> (w254:string)
        n111 = Concatenate Strings("Gain " ("string"), w244) -> (w252:string)
        n112 = Concatenate Strings("THD " ("string"), w246) -> (w253:string)
        n113 = property on="meas table" class="Tbl (strict)"() -> ("Column Headers[]"=w208:string[])  [unwired: 2 in, 2 out]
        n114 = Replace Array Subset(array=w208, new element #1=w255, index #1=5 ("index"), new element #2=w254, index #2=6 ("index"), new element #3=w253, index #3=7 ("index"), new element #4=w252, index #4=9 ("index")) -> (w256:string[])
        n115 = property on="meas table" class="Tbl (strict)"("Column Headers[]"=w256) -> ()  [unwired: 2 in, 2 out]
        n116 = local read "amplitude (Vrms)"() -> (w220:dbl[])
        n117 = local read "amplitude (dBFS)"() -> (w217:dbl[])
        n118 = local read "frequency (Hz)"() -> (w223:dbl[])
        n119 = local read "phase (deg)"() -> (w213:dbl[])
        n120 = local read "THD+N"() -> (w240:dbl[])
        n121 = local read "THD"() -> (w237:dbl[])
        n122 = local read "SNR"() -> (w242:dbl[])
        n123 = local read "channel names"() -> (w205:string[])
        n124 = for {
          tunnel: [w278] -> w222 mode=indexing
          tunnel: w223 -> [w277] mode=indexing
          tunnel: "%.3f" ("initial string") -> [w276]
          n125 = Format Into String(format string=w276, w277) -> (resulting string=w278:string)  [unwired: 2 in, 1 out]
        }
        n126 = for {
          tunnel: [w275] -> w219 mode=indexing
          tunnel: w220 -> [w274] mode=indexing
          tunnel: "%.3f" ("initial string") -> [w273]
          n127 = Format Into String(format string=w273, w274) -> (resulting string=w275:string)  [unwired: 2 in, 1 out]
        }
        n128 = for {
          tunnel: [w272] -> w216 mode=indexing
          tunnel: w217 -> [w271] mode=indexing
          tunnel: "%.3f" ("initial string") -> [w270]
          n129 = Format Into String(format string=w270, w271) -> (resulting string=w272:string)  [unwired: 2 in, 1 out]
        }
        n130 = for {
          tunnel: [w293] -> w236 mode=indexing
          tunnel: w237 -> [w292] mode=indexing
          tunnel: w235 -> [w291]
          n131 = Format Into String(format string=w291, w292) -> (resulting string=w293:string)  [unwired: 2 in, 1 out]
        }
        n132 = for {
          tunnel: [w299] -> w231 mode=indexing
          tunnel: w242 -> [w298] mode=indexing
          tunnel: w241 -> [w297]
          n133 = Format Into String(format string=w297, w298) -> (resulting string=w299:string)  [unwired: 2 in, 1 out]
        }
        n134 = for {
          tunnel: [w296] -> w239 mode=indexing
          tunnel: w240 -> [w295] mode=indexing
          tunnel: w238 -> [w294]
          n135 = Format Into String(format string=w294, w295) -> (resulting string=w296:string)  [unwired: 2 in, 1 out]
        }
        n136 = for {
          tunnel: [w269] -> w214 mode=indexing
          tunnel: w213 -> [w268] mode=indexing
          tunnel: "%.3f" ("initial string") -> [w267]
          n137 = Format Into String(format string=w267, w268) -> (resulting string=w269:string)  [unwired: 2 in, 1 out]
        }
        n138 = local read "dynamic range (dB)"() -> (w233:dbl[])
        n139 = local read "output power (W)"() -> (w229:dbl[])
        n140 = local read "SFDR (dBc)"() -> (w227:dbl[])
        n141 = local read "gain"() -> (w226:dbl[])
        n142 = for {
          tunnel: [w290] -> w232 mode=indexing
          tunnel: w233 -> [w289] mode=indexing
          tunnel: "%5.1f" ("initial string") -> [w288]
          n143 = Format Into String(format string=w288, w289) -> (resulting string=w290:string)  [unwired: 2 in, 1 out]
        }
        n144 = for {
          tunnel: [w281] -> w212 mode=indexing
          tunnel: w226 -> [w280] mode=indexing
          tunnel: w225 -> [w279]
          n145 = Format Into String(format string=w279, w280) -> (resulting string=w281:string)  [unwired: 2 in, 1 out]
        }
        n146 = for {
          tunnel: [w284] -> w211 mode=indexing
          tunnel: w227 -> [w283] mode=indexing
          tunnel: "%5.1f" ("initial string") -> [w282]
          n147 = Format Into String(format string=w282, w283) -> (resulting string=w284:string)  [unwired: 2 in, 1 out]
        }
        n148 = for {
          tunnel: [w287] -> w210 mode=indexing
          tunnel: w229 -> [w286] mode=indexing
          tunnel: "%.3f" ("initial string") -> [w285]
          n149 = Format Into String(format string=w285, w286) -> (resulting string=w287:string)  [unwired: 2 in, 1 out]
        }
        n150 = Build Array(w205, w222, w219, w216, w214, w231, w239, w236, w232, w212, w211, w210) -> (w209:string[][])
        n151 = Transpose 2D Array(2D array=w209) -> (transposed array=w206:string[][])
        "meas table" <- w206
        n152 = flat-sequence {
          tunnel: [w266] -> w207
          tunnel: w206 -> [_]
          tunnel: w203 -> [w264]
          frame #0 {
            n153 = control-ref of="meas table"() -> (w265:refnum<vi>)
            n154 = call "Autosize Columns (Table).vi"("error in (no error)"=w264, "table"=w265) -> ("error out"=w266:errorcluster)  [unwired: 9 in]
          }
        }
      }
      frame "Exit" {
        # "This case is triggered to close the User Interface from framework"
        n155 = Flush Queue(queue=w327, error in (no error)=w329) -> (queue out=w326:refnum<queue>, error out=w325:errorcluster)  [unwired: 1 out]
        n156 = Release Queue(queue=w326, force destroy? (F)=TRUE, error in (no error)=w325) -> (error out=w324:errorcluster)  [unwired: 2 out]
      }
      frame "Handle Error" {
      }
    }
  }
